vi "pressedButton.vi"(8 "error in (no error)":errorcluster, 10 "Bool Refnum":refnum<vi>, 11 "simonMessages in":refnum<class "simonMessages.lvclass">) -> (0 "error out":errorcluster, 3 "simonMessages out":refnum<class "simonMessages.lvclass">)   [LabVIEW 2019, in "simonMessages.lvclass"]
uses:
  simonMessages.lvclass
  simonMessages.lvclass/simonMessages.ctl
  TextDisplay/TextDisplay Class.lvclass
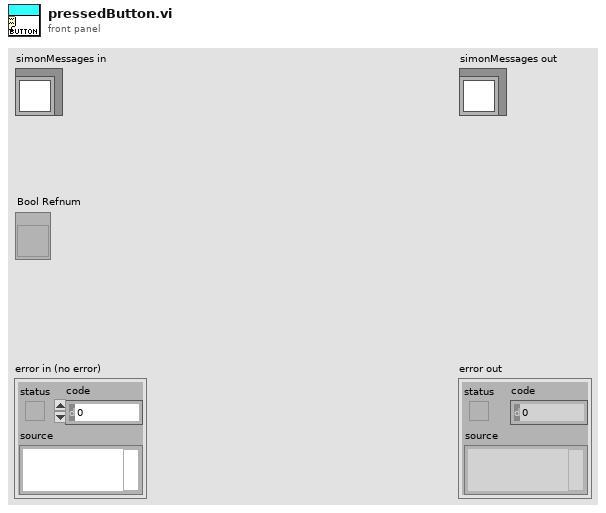
[diagram p1: front panel]
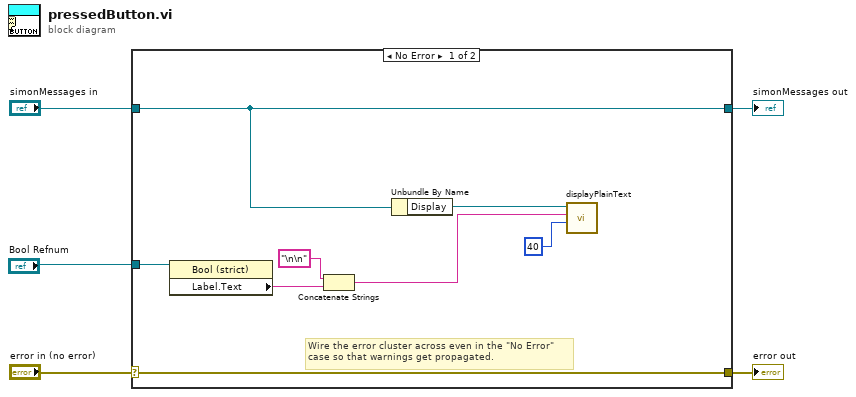
[diagram p0: block diagram]
diagram:
  n1 = case shown="No Error" "error in (no error)" {
    selector: "error in (no error)" -> [w13 w15]
    tunnel: [w13 w15] -> w4
    tunnel: [w10 w14] -> w2
    tunnel: "simonMessages in" -> [w10 w14]
    tunnel: "Bool Refnum" -> [w9 _]
    frame No Error {
      # "Wire the error cluster across even in the \"No Error\"\ncase so that warnings get propagated."
      n2 = property class="Bool (strict)"(reference=w9) -> ("Label.Text"=w8:string)  [unwired: 1 in, 2 out]
      n3 = Concatenate Strings("\n\n" ("string"), w8) -> (w7:string)
      n4 = Unbundle By Name(w10) -> ("Display"=w12:refnum<class "TextDisplay Class.lvclass">)
      n5 = call "displayPlainText.vi"("Font Size"=u32 40, "Text In"=w7, "TextDisplay Class in"=w12) -> ()  [unwired: 7 in, 2 out]
    }
    frame Error {
    }
  }
  "error out" <- w4
  "simonMessages out" <- w2
